vi "DesignPatterns_UpdateTreeControl.vi"(9 "Patterns":T6(array[cluster]), 10 "Tree Refnum":refnum<vi>, 11 "Panel":refnum<vi>) -> ()   [LabVIEW 2020]
uses:
  <resource>/Framework/Providers/Open_GDS/UML/DesignPattern/SubVIs/DesignPatterns_Pattern.ctl
  <resource>/Framework/Providers/Open_GDS/UML/DesignPattern/SubVIs/DesignPatterns_Node.ctl
  <resource>/Framework/Providers/Open_GDS/UML/DesignPattern/SubVIs/DesignPatterns_NodeType.ctl
  <resource>/Framework/Providers/Open_GDS/UML/DesignPattern/SubVIs/DesignPatterns_Link.ctl
  <resource>/Framework/Providers/Open_GDS/UML/DesignPattern/SubVIs/DesignPatterns_LinkType.ctl
  <vilib>/picture/picture.llb/imagedata.ctl
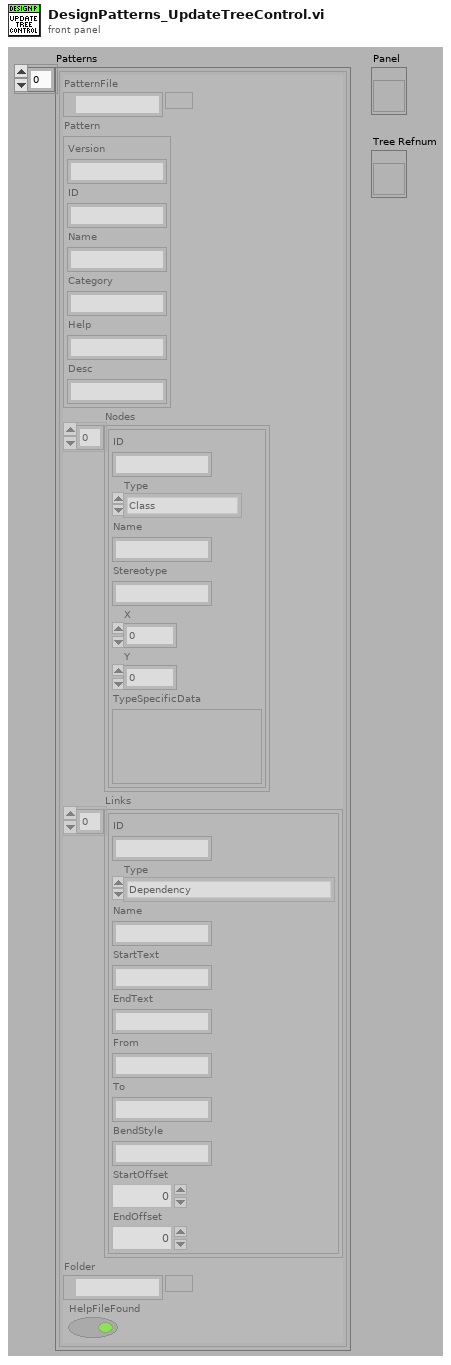
[diagram p1: front panel]
types:
  T1 = typedef "DesignPatterns_Pattern.ctl" = cluster{"Version":string, "ID":string, "Name":string, "Category":string, "Help":string, "Desc":string}
  T2 = typedef "DesignPatterns_Node.ctl" = cluster{"ID":string, "Type":T3, "Name":string, "Stereotype":string, "X":i32, "Y":i32, "TypeSpecificData":variant}
  T3 = typedef "DesignPatterns_NodeType.ctl" = enum16{"Class", "Interface", "Note", "Package"}
  T4 = typedef "DesignPatterns_Link.ctl" = cluster{"ID":string, "Type":T5, "Name":string, "StartText":string, "EndText":string, "From":string, "To":string, "BendStyle":string, "StartOffset":i32, "EndOffset":i32}
  T5 = typedef "DesignPatterns_LinkType.ctl" = enum16{"Dependency", "Inheritance", "Interface", "Association", "Aggregation", "CompositeAggregation"}
  T6 = cluster{"PatternFile":path, "Pattern":T1, "Nodes":T2[], "Links":T4[], "Folder":path, "HelpFileFound":bool}[]
  T7 = typedef "imagedata.ctl" = cluster{"image type":i32, "image depth":i32, "image":u8[], "mask":u8[], "colors":u32[], "Rectangle":cluster{"left":i16, "top":i16, "right":i16, "bottom":i16}}
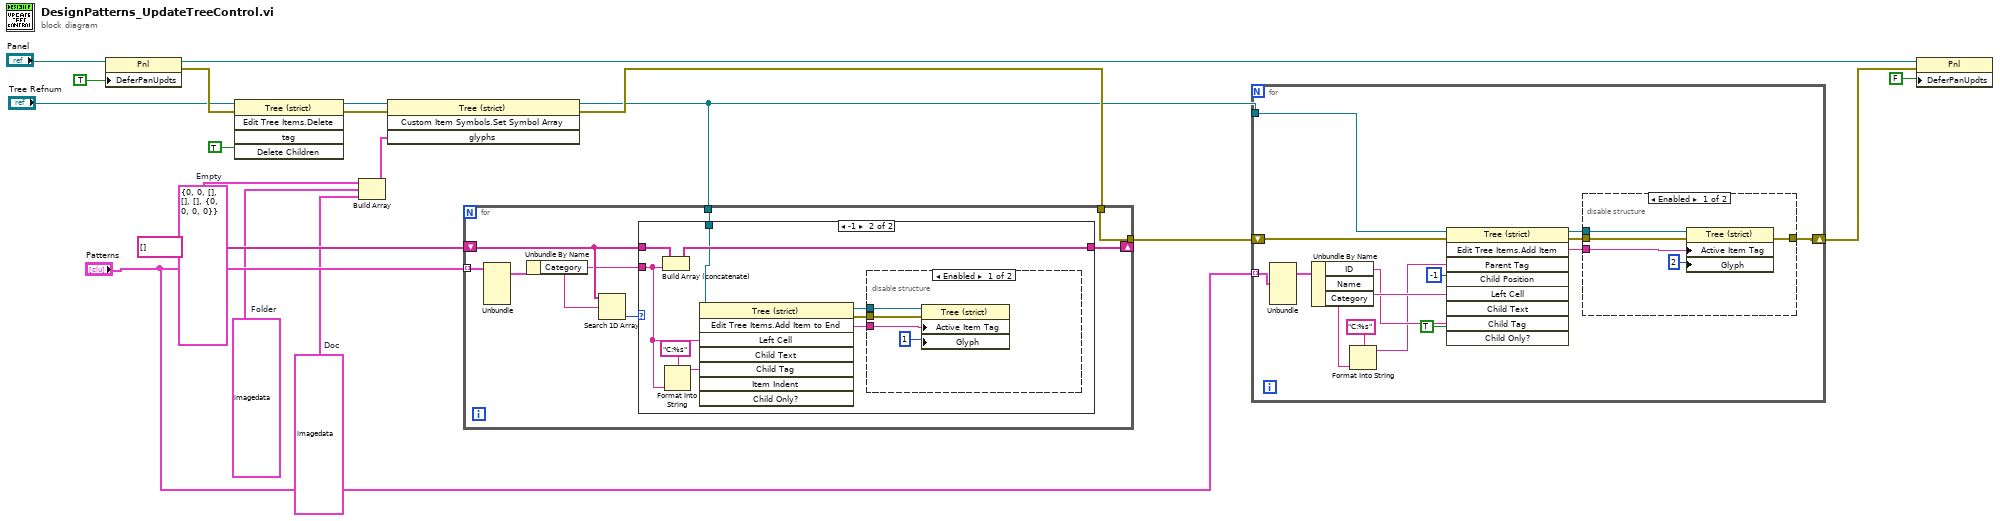
[diagram p0: block diagram]
diagram:
  w3 = T7 {"image type"=0, "image depth"=8, "image"=[30, 30, 30, 30, 30, 30, 30, 30, 30, 30, 30, 30, 30, 30, 30, 30, 30, 30, 30, 30, 30, 30, 30, 30, 30, 30, 30, 30, 30, 30, 30, 30, 30, 30, 30, 30, 30, 30, 30, 30, 30, 30, 30, 30, 30, 30, 30, 30, 30, 30, 11, 11, 9, 7, 7, 30, 30, 30, 30, 30, 30, 30, 30, 30, 30, 11, 30, 26, 26, 26, 24, 6, 5, 5, 4, 4, 4, 4, 30, 30, 30, 11, 30, 26, 26, 26, 24, 24, 24, 24, 21, 21, 24, 4, 30, 30, 30, 10, 29, 26, 26, 24, 5, 3, 3, 3, 2, 2, 1, 0, 30, 30, 30, 5, 5, 5, 5, 5, 28, 28, 28, 22, 22, 19, 23, 0, 30, 30, 30, 5, 29, 29, 29, 28, 17, 17, 16, 14, 14, 13, 22, 0, 30, 30, 30, 5, 27, 21, 21, 17, 17, 16, 14, 13, 12, 12, 19, 0, 30, 30, 30, 5, 25, 17, 17, 17, 16, 14, 13, 12, 8, 8, 18, 0, 30, 30, 30, 3, 23, 17, 17, 16, 14, 13, 12, 8, 6, 6, 15, 0, 30, 30, 30, 3, 23, 25, 25, 23, 22, 20, 19, 18, 15, 15, 20, 0, 30, 30, 30, 3, 2, 2, 2, 2, 2, 1, 1, 1, 1, 1, 1, 0, 30, 30, 30, 30, 30, 30, 30, 30, 30, 30, 30, 30, 30, 30, 30, 30, 30, 30, 30, 30, 30, 30, 30, 30, 30, 30, 30, 30, 30, 30, 30, 30, 30, 30], "mask"=[], "colors"=[15445554, 15446583, 15447613, 15449158, 15454001, 15451729, 15584873, 15453561, 15848822, 15454091, 15454604, 15455128, 15981443, 16179341, 16245911, 16180138, 16378273, 16576172, 16180912, 16313013, 16378557, 16708534, 16510659, 16643012, 16775109, 16577743, 16775118, 16774867, 16578536, 16776179, 16777215, 0, 0, 0, 0, 0, 0, 0, 0, 0, 0, 0, 0, 0, 0, 0, 0, 0, 0, 0, 0, 0, 0, 0, 0, 0, 0, 0, 0, 0, 0, 0, 0, 0, 0, 0, 0, 0, 0, 0, 0, 0, 0, 0, 0, 0, 0, 0, 0, 0, 0, 0, 0, 0, 0, 0, 0, 0, 0, 0, 0, 0, 0, 0, 0, 0, 0, 0, 0, 0, 0, 0, 0, 0, 0, 0, 0, 0, 0, 0, 0, 0, 0, 0, 0, 0, 0, 0, 0, 0, 0, 0, 0, 0, 0, 0, 0, 0, 0, 0, 0, 0, 0, 0, 0, 0, 0, 0, 0, 0, 0, 0, 0, 0, 0, 0, 0, 0, 0, 0, 0, 0, 0, 0, 0, 0, 0, 0, 0, 0, 0, 0, 0, 0, 0, 0, 0, 0, 0, 0, 0, 0, 0, 0, 0, 0, 0, 0, 0, 0, 0, 0, 0, 0, 0, 0, 0, 0, 0, 0, 0, 0, 0, 0, 0, 0, 0, 0, 0, 0, 0, 0, 0, 0, 0, 0, 0, 0, 0, 0, 0, 0, 0, 0, 0, 0, 0, 0, 0, 0, 0, 0, 0, 0, 0, 0, 0, 0, 0, 0, 0, 0, 0, 0, 0, 0, 0, 0, 0, 0, 0, 0, 0, 0, 0, 0, 0, 0, 0, 0, 0, 0, 0, 0, 0, 0], "Rectangle"={"left"=0, "top"=0, "right"=16, "bottom"=16}}  # Folder
  w4 = T7 {"image type"=0, "image depth"=0, "image"=[], "mask"=[], "colors"=[], "Rectangle"={"left"=0, "top"=0, "right"=0, "bottom"=0}}  # Empty
  w7 = T7 {"image type"=0, "image depth"=8, "image"=[31, 31, 31, 31, 31, 31, 31, 31, 31, 31, 31, 31, 31, 0, 0, 0, 31, 18, 16, 27, 22, 21, 21, 5, 5, 6, 6, 6, 6, 31, 0, 0, 31, 16, 18, 4, 2, 4, 2, 2, 4, 4, 4, 4, 14, 7, 31, 0, 31, 27, 4, 1, 1, 1, 1, 1, 19, 19, 19, 11, 14, 14, 7, 31, 31, 22, 11, 1, 1, 1, 1, 19, 19, 3, 3, 11, 11, 11, 15, 31, 31, 21, 11, 1, 1, 1, 19, 19, 19, 3, 12, 12, 20, 11, 15, 31, 31, 21, 11, 1, 1, 19, 19, 19, 3, 12, 12, 20, 9, 11, 15, 31, 31, 5, 11, 1, 19, 19, 3, 3, 12, 20, 20, 9, 9, 11, 10, 31, 31, 5, 11, 19, 19, 3, 12, 12, 20, 9, 9, 13, 13, 4, 10, 31, 31, 6, 2, 19, 19, 3, 12, 20, 9, 9, 13, 13, 29, 4, 17, 31, 31, 6, 2, 3, 3, 12, 20, 9, 9, 13, 13, 29, 29, 26, 17, 31, 31, 6, 2, 3, 12, 12, 20, 9, 13, 13, 29, 8, 8, 23, 25, 31, 31, 6, 11, 3, 12, 20, 9, 9, 13, 29, 29, 8, 8, 2, 25, 31, 31, 7, 30, 11, 2, 4, 4, 26, 26, 26, 26, 23, 2, 28, 24, 31, 31, 6, 7, 7, 7, 15, 15, 10, 10, 17, 17, 25, 25, 24, 15, 31, 31, 31, 31, 31, 31, 31, 31, 31, 31, 31, 31, 31, 31, 31, 31, 31], "mask"=[], "colors"=[0, 13100030, 15528438, 12311805, 15068661, 8957896, 7772084, 5730449, 9816828, 11261179, 4805995, 15922938, 11983612, 10801659, 9026540, 5398907, 11457509, 4410204, 14018544, 12640253, 11655164, 10141910, 11062238, 14608367, 2699587, 4080981, 14871024, 11588067, 13356241, 10407675, 14015460, 16777215, 0, 0, 0, 0, 0, 0, 0, 0, 0, 0, 0, 0, 0, 0, 0, 0, 0, 0, 0, 0, 0, 0, 0, 0, 0, 0, 0, 0, 0, 0, 0, 0, 0, 0, 0, 0, 0, 0, 0, 0, 0, 0, 0, 0, 0, 0, 0, 0, 0, 0, 0, 0, 0, 0, 0, 0, 0, 0, 0, 0, 0, 0, 0, 0, 0, 0, 0, 0, 0, 0, 0, 0, 0, 0, 0, 0, 0, 0, 0, 0, 0, 0, 0, 0, 0, 0, 0, 0, 0, 0, 0, 0, 0, 0, 0, 0, 0, 0, 0, 0, 0, 0, 0, 0, 0, 0, 0, 0, 0, 0, 0, 0, 0, 0, 0, 0, 0, 0, 0, 0, 0, 0, 0, 0, 0, 0, 0, 0, 0, 0, 0, 0, 0, 0, 0, 0, 0, 0, 0, 0, 0, 0, 0, 0, 0, 0, 0, 0, 0, 0, 0, 0, 0, 0, 0, 0, 0, 0, 0, 0, 0, 0, 0, 0, 0, 0, 0, 0, 0, 0, 0, 0, 0, 0, 0, 0, 0, 0, 0, 0, 0, 0, 0, 0, 0, 0, 0, 0, 0, 0, 0, 0, 0, 0, 0, 0, 0, 0, 0, 0, 0, 0, 0, 0, 0, 0, 0, 0, 0, 0, 0, 0, 0, 0, 0, 0, 0, 0, 0, 0, 0, 0, 0, 0], "Rectangle"={"left"=0, "top"=0, "right"=16, "bottom"=16}}  # Doc
  n1 = property class="Pnl"(reference="Panel", "DeferPanUpdts"=TRUE ("Defer Panel Updates")) -> (reference out=w19:refnum<vi>, error out=w11:errorcluster)  [unwired: 1 in]
  n2 = invoke on="Invoke Node" class="Tree (strict)" method="Edit Tree Items.Delete"(reference="Tree Refnum", error in=w11, "Delete Children"=TRUE ("Delete Children?")) -> (reference out=w10:refnum<vi>, error out=w5:errorcluster)  [unwired: 2 in, 3 out]
  n3 = Build Array(w4, w3, w7) -> (w6:T7[])
  n4 = invoke on="Invoke Node" class="Tree (strict)" method="Custom Item Symbols.Set Symbol Array"(reference=w10, error in=w5, "glyphs"=w6) -> (reference out=w8:refnum<vi>, error out=w9:errorcluster)  [unwired: 1 in, 2 out]
  n5 = for {
    tunnel: "Patterns" -> [w27] mode=indexing
    tunnel: w8 -> [w23]
    shift-right: [w26] -> _
    shift-left: string[] [] -> [w25]
    tunnel: w9 -> [w21]
    tunnel: [w21] -> w12
    n6 = Unbundle(w27) -> ("Pattern"=w20:T1)  [unwired: 5 out]
    n7 = Unbundle By Name(w20) -> ("Category"=w24:string)
    n8 = Search 1D Array(1D array=w25, element=w24) -> (index of element=w22:i32)  [unwired: 1 out]
    n9 = case shown="-1" w22 {
      tunnel: [w28 w37] -> w26
      tunnel: w25 -> [w28 w36]
      tunnel: w24 -> [_ w31]
      tunnel: w23 -> [_ w35]
      frame 0, Default {
      }
      frame -1 {
        n10 = Build Array (concatenate)(w36, w31) -> (w37:string[])
        n11 = Format Into String(format string="C:%s", w31) -> (resulting string=w30:string)  [unwired: 2 in, 1 out]
        n12 = invoke on="Invoke Node" class="Tree (strict)" method="Edit Tree Items.Add Item to End"(reference=w35, "Left Cell"=w31, "Child Tag"=w30) -> (reference out=w34:refnum<vi>, error out=w29:errorcluster, "Edit Tree Items:Add Item to End"=w33:string)  [unwired: 5 in, 5 out]
        n13 = disable-structure shown="Enabled" {
          disable-tunnel: w34 -> [w41 _]
          disable-tunnel: w33 -> [w40 _]
          disable-tunnel: w29 -> [w39 _]
          frame Enabled {
            n14 = property class="Tree (strict)"(reference=w41, error in=w39, "Active Item Tag"=w40, "Glyph"=1 ("Active Item:Symbol Index")) -> ()  [unwired: 2 out]
          }
          frame Disabled {
          }
        }
      }
    }
  }
  n15 = for {
    tunnel: w8 -> [w56]
    tunnel: "Patterns" -> [w55] mode=indexing
    shift-right: [w45] -> w13
    shift-left: w12 -> [w52]
    n16 = Unbundle(w55) -> ("Pattern"=w42:T1)  [unwired: 5 out]
    n17 = Unbundle By Name(w42) -> ("ID"=w51:string, "Name"=w54:string, "Category"=w49:string)
    n18 = Format Into String(format string="C:%s", w49) -> (resulting string=w48:string)  [unwired: 2 in, 1 out]
    n19 = invoke on="Invoke Node" class="Tree (strict)" method="Edit Tree Items.Add Item"(reference=w56, error in=w52, "Parent Tag"=w48, "Child Position"=-1, "Left Cell"=w54, "Child Tag"=w51, "Child Only?"=TRUE) -> (reference out=w47:refnum<vi>, error out=w44:errorcluster, "Edit Tree Items:Add Item"=w46:string)  [unwired: 2 in, 6 out]
    n20 = disable-structure shown="Enabled" {
      disable-tunnel: w47 -> [w58 _]
      disable-tunnel: w46 -> [w59 _]
      disable-tunnel: [w60 _] -> w45
      disable-tunnel: w44 -> [w57 _]
      frame Enabled {
        n21 = property class="Tree (strict)"(reference=w58, error in=w57, "Active Item Tag"=w59, "Glyph"=2 ("Active Item:Symbol Index")) -> (error out=w60:errorcluster)  [unwired: 1 out]
      }
      frame Disabled {
      }
    }
  }
  n22 = property class="Pnl"(reference=w19, error in=w13, "DeferPanUpdts"=FALSE ("Defer Panel Updates")) -> ()  [unwired: 2 out]
